vi "HFRR ADV v026 new software.vi"() -> ()   [LabVIEW 2025] (continued)
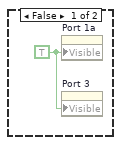
[diagram p3: hidden frame]
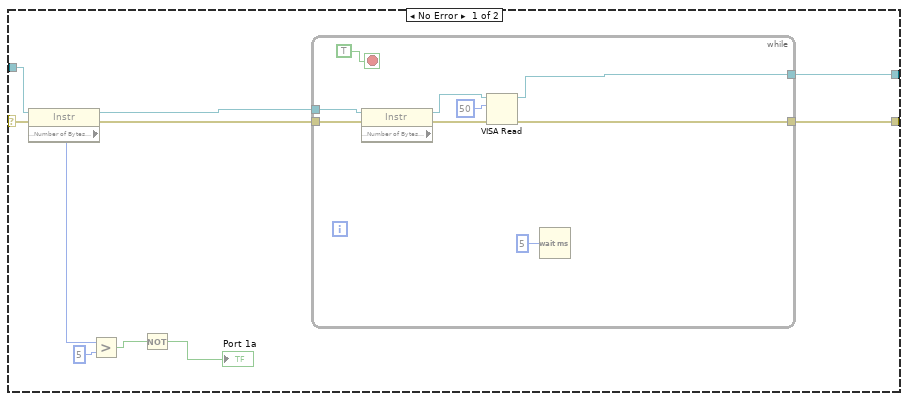
[diagram p4: hidden frame]
            n2893 = call-poly <vilib>:"Append Report Text.vi"("report in"=w3834, "error in (no error)"=w3833) -> ("report out"=w3855:refnum<class "NI_report.lvclass">, "error out"=w3853:errorcluster)  [unwired: 10 in, 2 out]
            n2894 = Concatenate Strings(w3809, w3808, w3807) -> (→"output":string)
            n2895 = call-poly <vilib>:"Append Report Text.vi"("report in"=w3855, "text"=w3808, "error in (no error)"=w3853) -> ("report out"=w3854:refnum<class "NI_report.lvclass">, "error out"=w3852:errorcluster)  [unwired: 9 in, 2 out]
            n2896 = call-dynamic "Print Report.vi"("report in"=w3854, "printer name (default)"=w3862, "error in (no error)"=w3852) -> ("report out"=w3864:refnum<class "NI_report.lvclass">, "error out"=w3865:errorcluster)  [unwired: 11 in]
            n2897 = call-dynamic "Dispose Report.vi"("report in"=w3864, "error in (no error)"=w3865) -> ()  [unwired: 13 in, 1 out]
          }
        }
        n2898 = case shown="True" "Print 2" {
          frame False {
          }
          frame True {
            n2899 = flat-sequence {
              frame #0 {
                n2900 = local read "s.NO"() -> (→"s.NO 2":string)
                n2901 = Wait (ms)(milliseconds to wait=u32 20) -> ()  [unwired: 1 out]
                n2902 = local read "Sample ID  3"() -> (→"Sample ID  6":string)
                n2903 = local read "Sample ID  4"() -> (→"Sample ID  7":string)
                n2904 = local read "Sample ID"() -> (→"Sample ID  2":string)
                n2905 = local read "Tested by"() -> (→"Tested by 2":string)
                n2906 = local read "Test Date"() -> (→"Test Date 2":string)
                n2907 = local read "Humidity after test 3"() -> (→"Humidity after test 4":dbl)
                n2908 = local read "Ref A Test Date :"() -> (→"TITTLE 4":string)
                n2909 = local read "Temperature before test 3"() -> (w3687:dbl)
                n2910 = local read "Temperature before test 3"() -> (→"Temperature after test 5":dbl)
                n2911 = local read "Temperature after test 3"() -> (→"Temperature after test 4":dbl)
                n2912 = local read "Humidity before test 3"() -> (→"Humidity before test 4":dbl)
                n2913 = local write "Temperature before test 3"(w3687) -> ()
                n2914 = local read "image data"() -> (w3678:T15)
                n2915 = String To Path(string="C:\\LAB-IQ\\im\\Temp_resized.jpg") -> (path=w3679:path)
                "path 2" <- w3679
                n2916 = call <vilib>:"Write JPEG File.vi"("image data"=w3678, "path to JPEG file"=w3679) -> ()  [unwired: 8 in, 2 out]
                "Ref A Test Date :" <- "Ref A Test Date :"
                "Ref B Test Date :" <- "Ref B Test Date :"
                "Ref B Scar Value :" <- "Ref B Scar Value :"
                "Ref A Scar Value :" <- "Ref A Scar Value :"
              }
              frame #1 {
                (unwired) HTML_Report_Image_Alignment."MIDDLE" ("alignment (default)")
                w3715 = u16 0 items=["portrait", "landscape"] ("orientation (portrait)")
                (unwired) HTML_Report_Image_Alignment."ABSMIDDLE" ("alignment (default)")
                (unwired) "TESTED BY : "
                (unwired) "TESTED DATE :"
                (unwired) "SAMPLE ID : "
                (unwired) "SAMPLE DESIGN : "
                w3748 = "\r"
                # "add image"
                n2917 = Wait (ms)(milliseconds to wait=u32 20) -> ()  [unwired: 1 out]
                n2918 = local read "Sample ID  2"() -> (w3741:string)
                n2919 = local read "Wear Scar X"() -> (w3713:dbl)
                "Length ( microns ) 2" <- w3713
                n2920 = local read "Wear Scar Y"() -> (w3712:dbl)
                "Wear Scar Y ( microns ) :" <- w3712
                n2921 = local read "Test Date 2"() -> (w3742:string)
                n2922 = local read "Tested by 2"() -> (w3743:string)
                n2923 = local read "String 46"() -> (w3739:string)
                n2924 = local read "String 48"() -> (w3745:string)
                n2925 = local read "String 47"() -> (w3744:string)
                n2926 = local read "String 49"() -> (w3746:string)
                n2927 = local read "String 10"() -> (w3699:string)
                n2928 = local read "s.NO 2"() -> (w3740:string)
                n2929 = Add(x=w3713, y=w3712) -> (x+y=w3711:dbl)
                n2930 = call <vilib>:"New Report.vi"("report type"=enum16{"Standard Report", "HTML"}."HTML") -> ("report out"=w3719:refnum<class "NI_report.lvclass">, "error out"=w3717:errorcluster)  [unwired: 13 in]
                n2931 = Concatenate Strings(w3748, w3739, w3740, w3748, w3745, w3741, w3748, w3744, w3742, w3748, w3746, w3743, w3748) -> (→"test by 2":string)
                n2932 = Concatenate Strings("C:\\LAB-IQ\\Data\\" ("string"), w3699, ".jpg" ("string")) -> ()  [unwired: 1 out]
                n2933 = Divide(x=w3711, y=2.0) -> (x/y=→"Mean Wear ( microns) :":dbl)
                n2934 = call-dynamic "Set Report Orientation.vi"("report in"=w3719, "orientation (portrait)"=w3715, "error in (no error)"=w3717) -> ("report out"=w3718:refnum<class "NI_report.lvclass">, "error out"=w3716:errorcluster)  [unwired: 11 in]
                n2935 = for {
                  N: 5 -> [_]
                  tunnel: w3718 -> [w3769]
                  tunnel: [w3768] -> w3697
                  tunnel: w3716 -> [w3767]
                  tunnel: [w3766] -> w3696
                  n2936 = call-dynamic "Set Report Tab Width.vi"("report in"=w3769, "error in (no error)"=w3767) -> ("report out"=w3768:refnum<class "NI_report.lvclass">, "error out"=w3766:errorcluster)  [unwired: 12 in]
                }
                n2937 = local read "TITTLE"() -> (w3714:string)
                n2938 = call-dynamic "Set Report Header Text.vi"("report in"=w3697, "center header text"=w3714, "error in (no error)"=w3696) -> ("report out"=w3735:refnum<class "NI_report.lvclass">, "error out"=w3734:errorcluster)  [unwired: 11 in]
                n2939 = for {
                  N: 1 -> [_]
                  tunnel: [w3773] -> w3721
                  tunnel: [w3772] -> w3720
                  tunnel: w3735 -> [w3771]
                  tunnel: w3734 -> [w3770]
                  n2940 = call-dynamic "New Report Line.vi"("report in"=w3771, "error in (no error)"=w3770) -> ("report out"=w3773:refnum<class "NI_report.lvclass">, "error out"=w3772:errorcluster)  [unwired: 12 in]
                }
                n2941 = for {
                  N: 2 -> [_]
                  tunnel: [w3765] -> w3727
                  tunnel: [w3764] -> w3726
                  tunnel: w3721 -> [w3763]
                  tunnel: w3720 -> [w3762]
                  n2942 = call-dynamic "New Report Line.vi"("report in"=w3763, "error in (no error)"=w3762) -> ("report out"=w3765:refnum<class "NI_report.lvclass">, "error out"=w3764:errorcluster)  [unwired: 12 in]
                }
                n2943 = for {
                  N: 25 -> [_]
                  tunnel: w3727 -> [w3761]
                  tunnel: w3726 -> [w3759]
                  tunnel: [w3760] -> w3730
                  tunnel: [w3758] -> w3729
                  n2944 = call-dynamic "Set Report Tab Width.vi"("report in"=w3761, "error in (no error)"=w3759) -> ("report out"=w3760:refnum<class "NI_report.lvclass">, "error out"=w3758:errorcluster)  [unwired: 12 in]
                }
                n2945 = control-ref of="Tab Control 9"() -> (w3725:refnum<vi>)
                n2946 = call-dynamic "Append Control Image to Report.vi"("report in"=w3730, "alignment (default)"=HTML_Report_Image_Alignment."ABSMIDDLE", "ctrl reference"=w3725, "error in (no error)"=w3729) -> ("report out"=w3724:refnum<class "NI_report.lvclass">, "error out"=w3723:errorcluster)  [unwired: 8 in, 2 out]
                n2947 = for {
                  N: 3 -> [_]
                  tunnel: [w3757] -> w3708
                  tunnel: [w3756] -> w3707
                  tunnel: w3724 -> [w3755]
                  tunnel: w3723 -> [w3754]
                  n2948 = call-dynamic "New Report Line.vi"("report in"=w3755, "error in (no error)"=w3754) -> ("report out"=w3757:refnum<class "NI_report.lvclass">, "error out"=w3756:errorcluster)  [unwired: 12 in]
                }
                n2949 = for {
                  N: 100 -> [_]
                  tunnel: w3708 -> [w3753]
                  tunnel: w3707 -> [w3751]
                  tunnel: [w3752] -> w3704
                  tunnel: [w3750] -> w3702
                  n2950 = call-dynamic "Set Report Tab Width.vi"("report in"=w3753, "error in (no error)"=w3751) -> ("report out"=w3752:refnum<class "NI_report.lvclass">, "error out"=w3750:errorcluster)  [unwired: 12 in]
                }
                n2951 = String To Path(string="C:\\LAB-IQ\\im\\Temp_resized.jpg") -> (path=w3694:path)
                n2952 = call-poly <vilib>:"Append Image to Report.vi"("report in"=w3704, "path or URL of image"=w3694, "error in (no error)"=w3702) -> ("report out"=w3703:refnum<class "NI_report.lvclass">, "error out"=w3701:errorcluster)  [unwired: 9 in, 2 out]
                n2953 = call-poly <vilib>:"Open HTML Report in Browser.vi"("report in"=w3703, "error in (no error)"=w3701) -> ("report out"=w3738:refnum<class "NI_report.lvclass">, "error out"=w3737:errorcluster)  [unwired: 11 in, 1 out]
                n2954 = call-dynamic "Dispose Report.vi"("report in"=w3738, "error in (no error)"=w3737) -> ()  [unwired: 13 in, 1 out]
              }
              frame #2 {
              }
              frame #3 {
                n2955 = disable-structure shown="Disabled" {
                  frame Disabled {
                    n2956 = local read "String 10"() -> (w3778:string)
                    n2957 = Concatenate Strings("C:\\LAB-IQ-NXT\\Data\\" ("string"), w3778, ".jpg" ("string")) -> (w3776:string)
                    n2958 = String To Path(string=w3776) -> (path=w3775:path)
                    n2959 = Delete(path (use dialog)=w3775) -> ()  [unwired: 4 in, 3 out]
                  }
                  frame Enabled {
                  }
                }
                n2960 = local write "Print 2"(FALSE ("Print")) -> ()
              }
            }
          }
        }
      }
    }
    n2961 = Wait (ms)(milliseconds to wait=u32 50) -> ()  [unwired: 1 out]
    n2962 = Wait (ms)(milliseconds to wait=u32 50) -> ()  [unwired: 1 out]
    n2963 = local read "Quit"() -> (w2123:bool)
  }
  n2964 = VISA Close(VISA resource name=w41, error in (no error)=w40) -> ()  [unwired: 1 out]
  n2965 = while {
    tunnel: [w3938] -> w49
    shift-right: [w3931] -> _
    shift-left: 0.0 -> [w3934]
    shift-right: [w3930] -> _
    shift-left: 0.0 -> [w3933]
    shift-right: [w3929] -> _
    shift-left: 100.0 ("vc_cmd") -> [w3932]
    stop <- w3938 stop-if-true
    # "PID LOGIC"
    n2966 = local read "RUN"() -> (w3936:bool)
    n2967 = local read "Auto Start Temp"() -> (w3925:bool)
    n2968 = local read "Auto Start Test"() -> (w3935:bool)
    n2969 = local read "START TEMP"() -> (w3927:bool)
    n2970 = And(x=w3925, y=w3935) -> (x .and. y?=w3926:bool)
    n2971 = Or(x=w3936, y=w3926) -> (x .or. y?=w3937:bool)
    n2972 = And(x=w3937, y=w3927) -> (x .and. y?=w3928:bool)
    n2973 = Wait (ms)(milliseconds to wait="milliseconds to wait") -> ()  [unwired: 1 out]
    n2974 = case shown="True" w3928 {
      tunnel: [400.0 ("out_vc_cmd") w3958] -> w3929
      tunnel: [w3941 w3960] -> w3930
      tunnel: [w3941 w3959] -> w3931
      tunnel: w3934 -> [_ w3949]
      tunnel: w3933 -> [_ w3948]
      tunnel: w3932 -> [_ w3947]
      frame False {
        w3941 = 0.0 ("error_out")
      }
      frame True {
        n2975 = local read "Set Strk"() -> (w3944:dbl)
        n2976 = local read "LVDT STROKE"() -> (w3942:dbl)
        n2977 = Add(x=w3944, y="Add up Stroke") -> (x+y=w3945:dbl)
        n2978 = formula code="// Zero-Hardcode Explicit Positional-Form PID Engine\n// Inputs: target_stroke, measured_stroke, dt, prev_error, integral_accumulator_in, prev_vc_cmd\n//         kp, ki, kd, max_step_change, max_amplitude, min_amplitude, startup_cmd\n// Outputs: vc_cmd, error_out, out_error, integral_accumulator_out, out_vc_cmd\n\n// 1. Calculate Tracking Error\nfloat current_error = target_stroke - measured_stroke;\nerror_out = current_error;\n\n// 2. Compute Proportional Term\nfloat p_term = kp * current_error;\n\n// 3. Compute Derivative Term\nfloat d_term = 0.0;\nif (dt > 0.0) {\n    d_term = kd * ((current_error - prev_error) / dt);\n}\n\n// 4. Update and Accumulate Integral Term\nfloat current_integral = integral_accumulator_in + (current_error * dt);\nfloat i_term = ki * current_integral;\n\n// 5. Calculate Ideal Target Command\nfloat ideal_command = startup_cmd + p_term + i_term + d_term;\n\n// 6. Anti-Windup Protection (Back-calculation method)\nif (ideal_command > max_amplitude) {\n    float excess = ideal_command - max_amplitude;\n    if (ki > 0.0) {\n        current_integral -= excess / ki;\n    }\n    ideal_command = max_amplitude;\n} else if (ideal_command < min_amplitude) {\n    float excess = ideal_command - min_amplitude;\n    if (ki > 0.0) {\n        current_integral -= excess / ki;\n    }\n    ideal_command = min_amplitude;\n}\n\n// 7. Apply Loop Rate Limiting (Protects voice coil from large voltage steps)\nfloat raw_adjustment = ideal_command - prev_vc_cmd;\n\nif (raw_adjustment > max_step_change) {\n    raw_adjustment = max_step_change;\n} else if (raw_adjustment < -max_step_change) {\n    raw_adjustment = -max_step_change;\n}\n\nfloat next_vc_cmd = prev_vc_cmd + raw_adjustment;\n\n// Final Output Safety Safeguard Clamping\nif (next_vc_cmd > max_amplitude) {\n    next_vc_cmd = max_amplitude;\n} else if (next_vc_cmd < min_amplitude) {\n    next_vc_cmd = min_amplitude;\n}\n\n// 8. Map to Shift Registers for memory persistence\nvc_cmd = next_vc_cmd;\nout_error = current_error;                     \nintegral_accumulator_out = current_integral;  \nout_vc_cmd = next_vc_cmd;"("target_stroke"=w3945, "measured_stroke"=w3942, "dt"="dt", "integral_accumulator_in"=w3948, "prev_error"=w3949, "prev_vc_cmd"=w3947, "kp"="kp", "ki"="ki", "kd"="kd", "max_step_change"="max_step_change", "max_amplitude"="max_amplitude", "min_amplitude"="min_amplitude", "startup_cmd"="startup_cmd") -> ("vc_cmd"=w3964:dbl, "out_error"=w3959:dbl, "integral_accumulator_out"=w3960:dbl, "out_vc_cmd"=w3958:dbl)  [unwired: 1 out]
        "output Vpp" <- w3964
        n2979 = Number To Fractional String(number=w3964, precision (6)=i16 1) -> (F-format string=w3962:string)  [unwired: 2 in]
        n2980 = Concatenate Strings("DAC;" ("string"), w3962) -> (w3946:string)
        n2981 = local write "Due Write"(w3946) -> ()
        "prev_error" <- w3949
        "integral_accumulator_in" <- w3948
        "prev_vc_cmd" <- w3947
      }
    }
    n2982 = local read "Quit"() -> (w3938:bool)
  }
  n2983 = Or(x=w45, y=w44) -> (x .or. y?=w46:bool)
  n2984 = Or(x=w42, y=w46) -> (x .or. y?=w51:bool)
  n2985 = control-ref of="new picture"() -> ()  [unwired: 1 out]
  n2986 = Or(x=w54, y=w51) -> (x .or. y?=w48:bool)
  n2987 = Or(x=w48, y=w49) -> (x .or. y?=w43:bool)
  n2988 = while {
    tunnel: [w3965] -> w53
    i -> [w3972]
    stop <- w3965 stop-if-true
    n2989 = local read "Quit"() -> (w3965:bool)
    n2990 = Equal To 0?(x=w3972) -> (x = 0?=w3970:bool)
    n2991 = call "Elapsed Time3"("Time Target (s)"=45.0, "Auto Reset"=TRUE) -> ("Time has Elapsed"=w3969:bool)  [unwired: 10 in, 7 out]
    n2992 = Wait (ms)(milliseconds to wait=u32 50) -> ()  [unwired: 1 out]
    n2993 = Or(x=w3969, y=w3970) -> (x .or. y?=w3971:bool)
    n2994 = case shown="True" w3971 {
      frame False {
      }
      frame True {
        n2995 = call <vilib>:"System Exec.vi"("run minimized? (F)"=TRUE, "error in (no error)"="error in (no error)", "command line"="powercfg.exe -change -monitor-timeout-ac 0") -> ("error out"=w3983:errorcluster)  [unwired: 5 in, 3 out]
        n2996 = call <vilib>:"System Exec.vi"("run minimized? (F)"=TRUE, "error in (no error)"=w3983, "command line"="powercfg.exe -change -disk-timeout-ac 0") -> ("error out"=w3982:errorcluster)  [unwired: 5 in, 3 out]
        n2997 = call <vilib>:"System Exec.vi"("run minimized? (F)"=TRUE, "error in (no error)"=w3982, "command line"="powercfg.exe -change -standby-timeout-ac 0") -> ("error out"=w3981:errorcluster)  [unwired: 5 in, 3 out]
        n2998 = call <vilib>:"System Exec.vi"("run minimized? (F)"=TRUE, "error in (no error)"=w3981, "command line"="powercfg.exe -change -hibernate-timeout-ac 0") -> ("error out"=w3980:errorcluster)  [unwired: 5 in, 3 out]
        n2999 = call <vilib>:"Simple Error Handler.vi"("error in (no error)"=w3980) -> ("error out"=w3986:errorcluster)  [unwired: 4 in, 4 out]
        n3000 = call <vilib>:"Clear Errors.vi"("error in (no error)"=w3986) -> ("error out"=→"error out":errorcluster)  [unwired: 5 in, 1 out]
      }
    }
  }
  n3001 = Compound Arithmetic op=OR(w56, w43, w53) -> (w55:bool)
  n3002 = flat-sequence {
    tunnel: w55 -> [_]
    tunnel: [w3988] -> w25
    tunnel: w25 -> [_]
    frame #0 {
      n3003 = call "CLOSE CONNECTION.vi"() -> ("error out"=w3988:errorcluster)  [unwired: 11 in]
    }
    frame #1 {
      n3004 = Quit LabVIEW(quit? (T)=TRUE) -> ()
      n3005 = local write "Quit"(FALSE ("EXIT")) -> ()
    }
  }
  n3006 = property on="Heater Button" class="Bool (strict)"("Visible"=TRUE) -> ()  [unwired: 2 in, 2 out]
  n3007 = while {
    tunnel: [w3995] -> _
    i -> [w3995]
    stop <- w3991 stop-if-true
    # "Langauage selection"
    n3008 = Equal?(x="Lan flag", y=22.0) -> ()  [unwired: 1 out]
    n3009 = disable-structure shown="Disabled" {
      frame Disabled {
        n3010 = stacked-sequence {
          frame #0 {
            n3011 = case shown="\"Russian\"" "Language Selection" {
              tunnel: [0 1] -> w3997
              frame "English", Default {
              }
              frame "Russian" {
              }
            }
            n3012 = for {
              N: 130 -> [_]
              tunnel: "Table" -> [w4006]
              tunnel: w3997 -> [w4005]
              i -> [w4004]
              n3013 = Index Array(array=w4006, index (row)=w4004, index (col)=w4005) -> (element=w4003:string)
              n3014 = case shown="1" w4004 {
                tunnel: w4003 -> [w4007 w4008 _ w4009 w4010 w4011 w4012 w4013 w4014 w4015 w4016 w4017 w4018 w4019 w4020 w4021 w4022 w4023 w4024 w4025 w4026 w4027 w4028 w4029 w4030 w4031 w4032 w4033 w4034 _ _ w4035 w4036 w4037 w4038 w4039 w4040 w4049 w4056 w4063 w4070 w4074 w4077 w4080 w4082 w4084 w4085 w4086 w4087 w4088 w4089 w4090 w4091 w4092 w4093 w4094 w4095 w4096 w4097 w4098 w4099 w4100 w4101 w4102 w4103 w4104 w4105 w4106 w4107 w4108 w4109 w4110 w4111 w4112 w4113 w4114 w4115 w4116 w4117 w4118 w4119 w4120 w4121 w4122 w4123 w4124 w4125 w4126 w4127 w4128 w4129 w4130 w4131 w4132 w4133 w4134 w4135 w4136 w4137 w4138 w4139 w4140 w4141 w4142 w4143 _ w4144 w4145 w4146 w4147 w4148 w4149 w4150 w4151 w4152 w4153 w4154 w4155 w4156 _ w4157 w4158 w4159 w4160 w4161 w4162 _]
                frame 0 {
                  n3015 = local write "S"(w4007) -> ()
                }
                frame 1 {
                  n3016 = local write "S 2"(w4008) -> ()
                }
                frame 2 {
                }
                frame 3 {
                  n3017 = local write "S 4"(w4009) -> ()
                }
                frame 4 {
                  n3018 = property on="FILE" class="Str"("Caption.Text"=w4010) -> ()  [unwired: 2 in, 2 out]
                }
                frame 5 {
                  n3019 = property on="Fuel Discription :" class="Str"("Caption.Text"=w4011) -> ()  [unwired: 2 in, 2 out]
                }
                frame 6 {
                  n3020 = property on="Remarks :" class="Str"("Caption.Text"=w4012) -> ()  [unwired: 2 in, 2 out]
                }
                frame 7 {
                  n3021 = property on="Save & Continue" class="Bool (strict)"("Boolean Text.Text"=w4013) -> ()  [unwired: 2 in, 2 out]
                }
                frame 8 {
                }
                frame 9 {
                  n3022 = property on="Set Hz" class="DigNum (strict)"("Caption.Text"=w4015) -> ()  [unwired: 2 in, 2 out]
                }
                frame 10 {
                }
                frame 11 {
                  n3023 = property on="NORMAL LOAD" class="DigNum (strict)"("Caption.Text"=w4017) -> ()  [unwired: 2 in, 2 out]
                }
                frame 12 {
                }
                frame 13 {
                  n3024 = property on="Set Temp" class="DigNum (strict)"("Caption.Text"=w4019) -> ()  [unwired: 2 in, 2 out]
                }
                frame 14 {
                  n3025 = local write "S 15"(w4020) -> ()
                }
                frame 15 {
                  n3026 = property on="Set Rh" class="DigNum (strict)"("Caption.Text"=w4021) -> ()  [unwired: 2 in, 2 out]
                }
                frame 16 {
                }
                frame 17 {
                  n3027 = local write "S 18"(w4023) -> ()
                }
                frame 18 {
                  "String 17" <- w4024
                }
                frame 19 {
                  n3028 = property on="test time" class="DigNum (strict)"("Caption.Text"=w4025) -> ()  [unwired: 2 in, 2 out]
                }
                frame 20 {
                  "String 18" <- w4026
                  "String 22" <- w4026
                }
                frame 21 {
                  n3029 = property on="Elapsed time" class="DigNum (strict)"("Caption.Text"=w4027) -> ()  [unwired: 2 in, 2 out]
                }
                frame 22 {
                  n3030 = property on="Samplingtime 2" class="DigNum (strict)"("Caption.Text"=w4028) -> ()  [unwired: 2 in, 2 out]
                }
                frame 23 {
                  "String 21" <- w4029
                }
                frame 24 {
                  n3031 = property on="Countdown" class="DigNum (strict)"("Caption.Text"=w4030) -> ()  [unwired: 2 in, 2 out]
                }
                frame 25 {
                  n3032 = property on="Countdown 2" class="DigNum (strict)"("Caption.Text"=w4031) -> ()  [unwired: 2 in, 2 out]
                }
                frame 26 {
                  n3033 = property on="Engage" class="Bool (strict)"("Boolean Text.Text"=w4032) -> ()  [unwired: 2 in, 2 out]
                }
                frame 27 {
                  n3034 = property on="Boolean  4" class="Bool (strict)"("Boolean Text.Text"=w4033) -> ()  [unwired: 2 in, 2 out]
                }
                frame 28 {
                  n3035 = property on="Test \nStatus" class="Bool (strict)"("Boolean Text.Text"=w4034) -> ()  [unwired: 2 in, 2 out]
                }
                frame 29 {
                }
                frame 30 {
                }
                frame 31 {
                }
                frame 32 {
                  n3036 = property on="RSTCOF" class="Bool"("Boolean Text.Text"=w4036) -> ()  [unwired: 2 in, 2 out]
                  n3037 = property on="RST FF" class="Bool"("Boolean Text.Text"=w4036) -> ()  [unwired: 2 in, 2 out]
                  n3038 = property on="RST TEMP" class="Bool"("Boolean Text.Text"=w4036) -> ()  [unwired: 2 in, 2 out]
                  n3039 = property on="RSTV1 3" class="Bool"("Boolean Text.Text"=w4036) -> ()  [unwired: 2 in, 2 out]
                  n3040 = property on="rstv2" class="Bool"("Boolean Text.Text"=w4036) -> ()  [unwired: 2 in, 2 out]
                  n3041 = property on="RSTV1 2" class="Bool"("Boolean Text.Text"=w4036) -> ()  [unwired: 2 in, 2 out]
                  n3042 = property on="RST CP" class="Bool"("Boolean Text.Text"=w4036) -> ()  [unwired: 2 in, 2 out]
                }
                frame 33 {
                  "S 61" <- w4037
                }
                frame 34 {
                  "String 23" <- w4038
                }
                frame 35 {
                  n3043 = property on="Rh Before" class="DigNum (strict)"("Caption.Text"=w4039) -> ()  [unwired: 2 in, 2 out]
                }
                frame 36 {
                  n3044 = Match Pattern(string=w4040, regular expression=",") -> (before substring=→"bs":string, after substring=→"as":string)  [unwired: 1 in, 2 out]
                  n3045 = property on="Rh After" class="DigNum (strict)"("Caption.Text"=w4040) -> ()  [unwired: 2 in, 2 out]
                }
                frame 37 {
                  n3046 = Match Pattern(string=w4049, regular expression=",") -> (before substring=w4048:string, after substring=w4047:string)  [unwired: 1 in, 2 out]
                  "bs" <- w4048
                  "as" <- w4047
                  n3047 = Concatenate Strings(w4048, w4047) -> (w4044:string)
                  n3048 = property on="Humidity before test 2" class="DigNum (strict)"("Caption.Text"=w4044) -> ()  [unwired: 2 in, 2 out]
                  n3049 = Concatenate Strings(w4044, "=" ("string")) -> (w4045:string)
                  n3050 = local write "S 38"(w4045) -> ()
                }
                frame 38 {
                  n3051 = Match Pattern(string=w4056, regular expression=",") -> (before substring=w4055:string, after substring=w4054:string)  [unwired: 1 in, 2 out]
                  "bs" <- w4055
                  "as" <- w4054
                  n3052 = Concatenate Strings(w4055, w4054) -> (w4051:string)
                  n3053 = property on="Humidity after test 2" class="DigNum (strict)"("Caption.Text"=w4051) -> ()  [unwired: 2 in, 2 out]
                  n3054 = Concatenate Strings(w4051, "=" ("string")) -> (w4053:string)
                  n3055 = local write "S 39"(w4053) -> ()
                }
                frame 39 {
                  n3056 = Match Pattern(string=w4063, regular expression=",") -> (before substring=w4062:string, after substring=w4061:string)  [unwired: 1 in, 2 out]
                  "bs" <- w4062
                  "as" <- w4061
                  n3057 = Concatenate Strings(w4062, w4061) -> (w4058:string)
                  n3058 = property on="Temperature before test 2" class="DigNum (strict)"("Caption.Text"=w4058) -> ()  [unwired: 2 in, 2 out]
                  n3059 = Concatenate Strings(w4058, "=" ("string")) -> (→"String 34":string)
                }
                frame 40 {
                  n3060 = Match Pattern(string=w4070, regular expression=",") -> (before substring=w4069:string, after substring=w4068:string)  [unwired: 1 in, 2 out]
                  "bs" <- w4069
                  "as" <- w4068
                  n3061 = Concatenate Strings(w4069, w4068) -> (w4065:string)
                  n3062 = property on="Temperature after test 2" class="DigNum (strict)"("Caption.Text"=w4065) -> ()  [unwired: 2 in, 2 out]
                  n3063 = Concatenate Strings(w4065, "=" ("string")) -> (→"String 35":string)
                  n3064 = property on="Temperature after test" class="DigNum (strict)"("Caption.Text"=w4065) -> ()  [unwired: 2 in, 2 out]
                }
                frame 41 {
                  n3065 = property on="AVP 2" class="DigNum (strict)"("Caption.Text"=w4074) -> ()  [unwired: 2 in, 2 out]
                  n3066 = Concatenate Strings(w4074, "=" ("string")) -> (→"String 36":string)
                }
                frame 42 {
                  n3067 = property on="MWSD 2" class="DigNum (strict)"("Caption.Text"=w4077) -> ()  [unwired: 2 in, 2 out]
                  n3068 = Concatenate Strings(w4077, "=" ("string")) -> (→"String 37":string)
                }
                frame 43 {
                  n3069 = property on="HCF 2" class="DigNum (strict)"("Caption.Text"=w4080) -> ()  [unwired: 2 in, 2 out]
                  n3070 = Concatenate Strings(w4080, "=" ("string")) -> (→"String 38":string)
                }
                frame 44 {
                  n3071 = Concatenate Strings(w4082, "=" ("string")) -> (→"String 39":string)
                  n3072 = property on="WS1.4 2" class="DigNum (strict)"("Caption.Text"=w4082) -> ()  [unwired: 2 in, 2 out]
                }
                frame 45 {
                }
                frame 46 {
                  n3073 = local write "S 47"(w4085) -> ()
                }
                frame 47 {
                  n3074 = local write "S 48"(w4086) -> ()
                }
                frame 48 {
                  n3075 = local write "S 49"(w4087) -> ()
                }
                frame 49 {
                  n3076 = local write "S 50"(w4088) -> ()
                }
                frame 50 {
                  n3077 = local write "S 51"(w4089) -> ()
                }
                frame 51 {
                  n3078 = local write "S 52"(w4090) -> ()
                }
                frame 52 {
                  n3079 = local write "S 53"(w4091) -> ()
                }
                frame 53 {
                  n3080 = local write "S 54"(w4092) -> ()
                }
                frame 54 {
                  n3081 = local write "S 55"(w4093) -> ()
                }
                frame 55 {
                  n3082 = local write "S 56"(w4094) -> ()
                }
                frame 56 {
                  n3083 = local write "S 57"(w4095) -> ()
                }
                frame 57 {
                  n3084 = local write "S 58"(w4096) -> ()
                }
                frame 58 {
                  n3085 = local write "S 59"(w4097) -> ()
                }
                frame 59 {
                  n3086 = local write "S 60"(w4098) -> ()
                }
                frame 60 {
                  n3087 = local write "S 62"(w4099) -> ()
                }
                frame 61 {
                  n3088 = local write "S 63"(w4100) -> ()
                }
                frame 62 {
                  n3089 = local write "S 64"(w4101) -> ()
                }
                frame 63 {
                  n3090 = local write "S 65"(w4102) -> ()
                }
                frame 64 {
                  n3091 = local write "S 66"(w4103) -> ()
                }
                frame 65 {
                  n3092 = local write "S 67"(w4104) -> ()
                }
                frame 66 {
                  n3093 = local write "S 68"(w4105) -> ()
                }
                frame 67 {
                  n3094 = local write "S 69"(w4106) -> ()
                }
                frame 68 {
                  n3095 = local write "S 70"(w4107) -> ()
                }
                frame 69 {
                  n3096 = local write "S 71"(w4108) -> ()
                }
                frame 70 {
                  n3097 = local write "S 72"(w4109) -> ()
                }
                frame 71 {
                  n3098 = local write "S 73"(w4110) -> ()
                }
                frame 72 {
                  n3099 = local write "S 74"(w4111) -> ()
                }
                frame 73 {
                  n3100 = local write "S 75"(w4112) -> ()
                }
                frame 74 {
                  n3101 = local write "S 76"(w4113) -> ()
                }
                frame 75 {
                  n3102 = local write "S 77"(w4114) -> ()
                }
                frame 76 {
                  n3103 = local write "S 78"(w4115) -> ()
                }
                frame 77 {
                  n3104 = local write "S 79"(w4116) -> ()
                }
                frame 79 {
                  n3105 = property on="Sample Temperature ( °C )" class="XYGraph (strict)"("Y Scale.Name Label.Text"=w4117) -> ()  [unwired: 2 in, 2 out]
                }
                frame 80 {
                  n3106 = local write "S 81"(w4118) -> ()
                  n3107 = property on="Humidity ( %RH )" class="XYGraph (strict)"("Y Scale.Name Label.Text"=w4118) -> ()  [unwired: 2 in, 2 out]
                }
                frame 78 {
                  n3108 = property on="Air Temperature  ( °C )" class="XYGraph (strict)"("X Scale.Name Label.Text"=w4119) -> ()  [unwired: 2 in, 2 out]
                  n3109 = property on="Humidity ( %RH )" class="XYGraph (strict)"("X Scale.Name Label.Text"=w4119) -> ()  [unwired: 2 in, 2 out]
                  n3110 = property on="Sample Temperature ( °C )" class="XYGraph (strict)"("X Scale.Name Label.Text"=w4119) -> ()  [unwired: 2 in, 2 out]
                  n3111 = property on="Coefficient Of Friction" class="XYGraph (strict)"("X Scale.Name Label.Text"=w4119) -> ()  [unwired: 2 in, 2 out]
                }
                frame 81 {
                  n3112 = property on="Air Temperature  ( °C )" class="XYGraph (strict)"("Y Scale.Name Label.Text"=w4120) -> ()  [unwired: 2 in, 2 out]
                }
                frame 82 {
                  n3113 = local write "S 84"(w4121) -> ()
                }
                frame 83 {
                  n3114 = local write "S 85"(w4122) -> ()
                }
                frame 84 {
                  n3115 = local write "S 86"(w4123) -> ()
                }
                frame 85 {
                  n3116 = local write "S 87"(w4124) -> ()
                }
                frame 86 {
                  n3117 = local write "S 88"(w4125) -> ()
                }
                frame 87 {
                }
                frame 88 {
                  n3118 = local write "S 90"(w4127) -> ()
                }
                frame 89 {
                  n3119 = local write "S 91"(w4128) -> ()
                }
                frame 90 {
                  n3120 = local write "S 92"(w4129) -> ()
                }
                frame 91 {
                  n3121 = local write "S 93"(w4130) -> ()
                }
                frame 92 {
                  n3122 = local write "S 94"(w4131) -> ()
                }
                frame 93 {
                  n3123 = local write "S 95"(w4132) -> ()
                }
                frame 94 {
                  n3124 = local write "S 96"(w4133) -> ()
                }
                frame 95 {
                  n3125 = local write "S 97"(w4134) -> ()
                }
                frame 96 {
                  n3126 = local write "S 98"(w4135) -> ()
                }
                frame 97 {
                  n3127 = local write "S 99"(w4136) -> ()
                }
                frame 98 {
                  n3128 = local write "S 100"(w4137) -> ()
                }
                frame 99 {
                  n3129 = local write "S 101"(w4138) -> ()
                }
                frame 100 {
                  n3130 = local write "S 102"(w4139) -> ()
                }
                frame 101 {
                  n3131 = local write "S 103"(w4140) -> ()
                }
                frame 102 {
                  n3132 = local write "S 104"(w4141) -> ()
                }
                frame 103 {
                  n3133 = local write "S 105"(w4142) -> ()
                }
                frame 104 {
                  n3134 = local write "S 106"(w4143) -> ()
                }
                frame 105 {
                }
                frame 106 {
                  n3135 = property on="OK Button 17" class="Bool (strict)"("Boolean Text.Text"=w4144) -> ()  [unwired: 2 in, 2 out]
                }
                frame 107 {
                  n3136 = property on="OK Button 16" class="Bool (strict)"("Boolean Text.Text"=w4145) -> ()  [unwired: 2 in, 2 out]
                }
                frame 108 {
                  n3137 = property on="TITTLE" class="Str"("Caption.Text"=w4146) -> ()  [unwired: 2 in, 2 out]
                }
                frame 109 {
                  "String 30" <- w4147
                }
                frame 110 {
                  n3138 = property on="Test Date" class="Str"("Caption.Text"=w4148) -> ()  [unwired: 2 in, 2 out]
                  "String 31" <- w4148
                }
                frame 111 {
                  n3139 = property on="Sample ID" class="Str"("Caption.Text"=w4149) -> ()  [unwired: 2 in, 2 out]
                  "String 32" <- w4149
                }
                frame 112 {
                  n3140 = property on="Tested by" class="Str"("Caption.Text"=w4150) -> ()  [unwired: 2 in, 2 out]
                  "String 33" <- w4150
                }
                frame 113 {
                  n3141 = property on="System Configured Printers 2" class="Arr (strict)"("Caption.Text"=w4151) -> ()  [unwired: 2 in, 2 out]
                }
                frame 114 {
                  n3142 = property on="Selected Printer" class="Str"("Caption.Text"=w4152) -> ()  [unwired: 2 in, 2 out]
                }
                frame 115 {
                  n3143 = property on="Select Printer 3" class="DigNum (strict)"("Caption.Text"=w4153) -> ()  [unwired: 2 in, 2 out]
                }
                frame 116 {
                  n3144 = property on="Print" class="Bool (strict)"("Boolean Text.Text"=w4154) -> ()  [unwired: 2 in, 2 out]
                }
                frame 117 {
                  "String 41" <- w4155
                }
                frame 118 {
                  n3145 = property on="tested by" class="Str"("Caption.Text"=w4156) -> ()  [unwired: 2 in, 2 out]
                }
                frame 119 {
                }
                frame 120 {
                  n3146 = property on="Export" class="Bool (strict)"("Boolean Text.Text"=w4157) -> ()  [unwired: 2 in, 2 out]
                }
                frame 121 {
                }
                frame 122 {
                }
                frame 123 {
                  n3147 = property on="Select File Type" class="Enum (strict)"("Caption.Text"=w4160) -> ()  [unwired: 2 in, 2 out]
                }
                frame 124 {
                  n3148 = property on="s.NO" class="Str"("Caption.Text"=w4161) -> ()  [unwired: 2 in, 2 out]
                  "String 45" <- w4161
                }
                frame 125 {
                  n3149 = property on="trip1 8" class="Bool (strict)"("Boolean Text.Text"=w4162) -> ()  [unwired: 2 in, 2 out]
                }
                frame 126, Default {
                }
              }
            }
          }
          frame #1 {
            w4170 = TRUE ("Visible")
            n3150 = local read "S 91"() -> (w4187:string)
            n3151 = local read "S 90"() -> (w4186:string)
            n3152 = local read "S 88"() -> (w4185:string)
            n3153 = property on="File Path" class="Path"("Caption.Text"=w4186) -> ()  [unwired: 2 in, 2 out]
            n3154 = local read "S 71"() -> (w4180:string)
            n3155 = local read "S 86"() -> (w4182:string)
            n3156 = local read "S 85"() -> (w4183:string)
            n3157 = local read "S 87"() -> (w4181:string)
            n3158 = local read "S 84"() -> (w4184:string)
            n3159 = local read "S 103"() -> (w4169:string)
            n3160 = local read "S 104"() -> (w4168:string)
            n3161 = property on="Password" class="Str"("Caption.Text"=w4183) -> ()  [unwired: 2 in, 2 out]
            n3162 = property on="EDIT" class="Bool (strict)"("Boolean Text.Text"=w4180) -> ()  [unwired: 2 in, 2 out]
            n3163 = property on="SAVE" class="Bool (strict)"("Boolean Text.Text"=w4184) -> ()  [unwired: 2 in, 2 out]
            n3164 = Build Array(w4169, w4168) -> (w4167:string[])
            n3165 = property on="Heater Button" class="Bool (strict)"("Strings [4]"=w4167) -> ()  [unwired: 2 in, 2 out]
            n3166 = local read "S 92"() -> (w4179:string)
            n3167 = local read "S 93"() -> (w4178:string)
            n3168 = local read "S 105"() -> (w4165:string)
            n3169 = local read "S 106"() -> (w4164:string)
            n3170 = Build Array(w4179, w4178) -> ()  [unwired: 1 out]
            n3171 = Build Array(w4165, w4164) -> (w4166:string[])
            n3172 = local read "S 95"() -> (w4176:string)
            n3173 = local read "S 94"() -> (w4177:string)
            n3174 = local read "bs"() -> (w4192:string)
            n3175 = local read "as"() -> (w4193:string)
            n3176 = property on="Humidity" class="Bool (strict)"("Strings [4]"=w4166) -> ()  [unwired: 2 in, 2 out]
            n3177 = Concatenate Strings(w4192, "\r", w4193) -> ()  [unwired: 1 out]
            n3178 = property on="Rh After" class="DigNum (strict)"("Caption.Size to Text?"=TRUE ("Caption.Size to Text")) -> ()  [unwired: 2 in, 2 out]
            n3179 = local read "S 48"() -> (w4216:string)
            n3180 = local read "S 50"() -> (w4214:string)
            n3181 = local read "S 51"() -> (w4213:string)
            n3182 = local read "S 49"() -> (w4215:string)
            n3183 = local read "S 52"() -> (w4212:string)
            n3184 = local read "as"() -> (w4197:string)
            n3185 = local read "bs"() -> (w4198:string)
            n3186 = local read "S 56"() -> (w4211:string)
            n3187 = local read "S 57"() -> (w4210:string)
            n3188 = local read "S 58"() -> (w4209:string)
            n3189 = local read "S 59"() -> (w4208:string)
            n3190 = property on="OPEN" class="Bool (strict)"("Boolean Text.Text"=w4212) -> ()  [unwired: 2 in, 2 out]
            n3191 = property on="OPEN 1" class="Bool (strict)"("Boolean Text.Text"=w4216) -> ()  [unwired: 2 in, 2 out]
            n3192 = property on="OPEN 2" class="Bool (strict)"("Boolean Text.Text"=w4215) -> ()  [unwired: 2 in, 2 out]
            n3193 = property on="OPEN 3" class="Bool (strict)"("Boolean Text.Text"=w4214) -> ()  [unwired: 2 in, 2 out]
            n3194 = property on="OPEN 4" class="Bool (strict)"("Boolean Text.Text"=w4213) -> ()  [unwired: 2 in, 2 out]
            n3195 = Concatenate Strings(w4198, "\r", w4197) -> ()  [unwired: 1 out]
            n3196 = local read "S 102"() -> (w4171:string)
            n3197 = property on="КОФ1" class="DigNum (strict)"("Caption.Text"=w4211) -> ()  [unwired: 2 in, 2 out]
            n3198 = local read "S 98"() -> (w4175:string)
            n3199 = local read "S 99"() -> (w4174:string)
            n3200 = local read "S 100"() -> (w4173:string)
            n3201 = local read "S 101"() -> (w4172:string)
            n3202 = property on="КОФ2" class="DigNum (strict)"("Caption.Text"=w4210) -> ()  [unwired: 2 in, 2 out]
            n3203 = property on="КОФ3" class="DigNum (strict)"("Caption.Text"=w4209) -> ()  [unwired: 2 in, 2 out]
            n3204 = property on="КОФ4" class="DigNum (strict)"("Caption.Text"=w4208) -> ()  [unwired: 2 in, 2 out]
            n3205 = local read "bs"() -> (w4196:string)
            n3206 = local read "as"() -> (w4195:string)
            n3207 = local read "S 60"() -> (w4207:string)
            n3208 = local read "S 54"() -> (w4217:string)
            n3209 = Concatenate Strings(w4196, "\r", w4195) -> ()  [unwired: 1 out]
            n3210 = Concatenate Strings(w4217, w4207) -> ()  [unwired: 1 out]
            n3211 = local read "S 77"() -> (→"String 43":string)
            n3212 = local read "S 76"() -> (w4190:string)
            n3213 = local read "S 78"() -> (w4189:string)
            n3214 = local read "S 71"() -> (w4201:string)
            n3215 = local read "S 66"() -> (w4206:string)
            n3216 = local read "S 67"() -> (w4205:string)
            n3217 = local read "S 68"() -> (w4204:string)
            n3218 = local read "S 69"() -> (w4203:string)
            n3219 = local read "S 70"() -> (w4202:string)
            n3220 = property on="AIR TEMP" class="DigNum (strict)"("Caption.Text"=w4189) -> ()  [unwired: 2 in, 2 out]
            n3221 = property on="Set Strk" class="DigNum (strict)"("Caption.Text"=w4190) -> ()  [unwired: 2 in, 2 out]
            n3222 = property on="SPEED OUT:" class="DigNum (strict)"("Caption.Text"=w4204) -> ()  [unwired: 2 in, 2 out]
            n3223 = property on="EDIT" class="Bool (strict)"("Boolean Text.Text"=w4201) -> ()  [unwired: 2 in, 2 out]
            n3224 = local read "S 79"() -> (w4188:string)
          }
          frame #2 {
          }
        }
        n3225 = local write "Lan flag"(10.0 ("Lan flag")) -> ()
      }
      frame Enabled {
      }
    }
    n3226 = Wait (ms)(milliseconds to wait=u32 2000) -> ()  [unwired: 1 out]
    n3227 = local read "Quit"() -> (w3991:bool)
  }
  n3228 = while {
    shift-right: [w4223] -> _
    shift-left: _ -> [w4224]
    shift-right: [w4221] -> _
    shift-left: T17 {"Read Heave and Surge"="", "Bytes at Heave Port"=0.0, "Heave and Surge COM Port:"="COM9", "Com Port 2"="COM7", "Residual Due"="", "Heave COM Status 2"=TRUE, "Heave COM Status"=TRUE, "Port 2"=TRUE, "Sway PPR"=6400.0, "Surge PPR"=6400.0, "Heave PPR"=6400.0, "Sway Pitch"=2.0, "Surge Pitch"=3.0, "Heave Pitch"=4.0, "Sway Pulses/mm"=320.0, "Surge Pulses/mm"=1600.0, "Heave Pulses/mm"=1600.0, "inner loop"=0.0, "Read Heave and Surge 2"="", "String 36"="", "Write S"=FALSE, "WriteCC1"=[""], "Heave COM Loop"=0, "LastCom"="", "EXIT"=FALSE, "Error Heave"={"status"=TRUE, "code"=-1073807343, "source"=""}} -> [w4220]
    shift-right: [w4218] -> _
    shift-left: enum16{"init", "MAIN", "Panel Close"}."init" -> [w4219]
    stop <- w4222 stop-if-true
    # "HUMIDITY LOOP LOGIC"
    n3229 = case shown="\"MAIN\"" w4219 {
      tunnel: w4224 -> [w4238 w4255 w4312 w4314]
      tunnel: [w4233 w4260 w4312 w4314] -> w4223
      tunnel: [_ _ TRUE _] -> w4222
      tunnel: [w4230 w4258 w4310 w4313] -> w4221
      tunnel: w4220 -> [w4235 w4254 w4310 w4313]
      tunnel: [enum16{"init", "MAIN", "Panel Close"}."MAIN" w4249 _ _] -> w4218
      frame "init" {
        n3230 = local read "Com Port 1"() -> (w4227:refnum<visa-resource-name>)
        n3231 = Bundle By Name(cluster=w4235, "Heave and Surge COM Port:"=w4227) -> (w4234:T17)
        n3232 = call "Instrument fgv uno.vi"("Enum"=T28."INIT", "error in (no error) 2"=w4238, "INPUT"=w4234) -> ("error"=w4236:errorcluster, "output"=w4232:T17)  [unwired: 6 in, 1 out]
        n3233 = case shown="Error" w4236 {
          selector: w4236 -> [w4240 _]
          tunnel: [w4240 w4244] -> w4233
          tunnel: w4232 -> [w4239 w4242]
          tunnel: [w4239 w4241] -> w4231
          frame No Error {
          }
          frame Error {
            n3234 = call "Instrument fgv uno.vi"("Enum"=T28."ERROR INIT", "INPUT"=w4242) -> ("error"=w4245:errorcluster, "output"=w4241:T17)  [unwired: 7 in, 1 out]
            n3235 = call <vilib>:"Clear Errors.vi"("error in (no error)"=w4245) -> ("error out"=w4244:errorcluster)  [unwired: 5 in, 1 out]
          }
        }
        n3236 = local read "LastCom Humidity"() -> (w4226:string)
        n3237 = Unbundle By Name(w4231) -> ("Heave COM Status 2"=→"COM Status":bool, "Error Heave"=→"Error  2":errorcluster)  [unwired: 1 out]
        n3238 = Bundle By Name(cluster=w4231, "LastCom"=w4226) -> (w4230:T17)
      }
      frame "MAIN" {
        n3239 = Unbundle By Name(w4254) -> ("Com Port 2"=w4262:refnum<visa-resource-name>)
        n3240 = local read "Com Port 1"() -> (w4248:refnum<visa-resource-name>)
        n3241 = local write "Com Port 5"(w4262) -> ()
        n3242 = Bundle By Name(cluster=w4254, "Heave and Surge COM Port:"=w4248) -> (w4253:T17)
        n3243 = Equal?(x=w4262, y=w4248) -> (x = y?=w4261:bool)
        n3244 = case shown="True" w4261 {
          tunnel: [w4266 w4283] -> w4260
          tunnel: w4255 -> [w4267 w4289]
          tunnel: w4253 -> [w4265 w4287]
          tunnel: [w4264 w4282] -> w4258
          frame False {
            n3245 = call <vilib>:"Clear Errors.vi"("error in (no error)"=w4267) -> ("error out"=w4263:errorcluster)  [unwired: 5 in, 1 out]
            n3246 = call "Instrument fgv uno.vi"("Enum"=T28."ERROR INIT", "error in (no error) 2"=w4263, "INPUT"=w4265) -> ("error"=w4269:errorcluster, "output"=w4264:T17)  [unwired: 6 in, 1 out]
            n3247 = call <vilib>:"Clear Errors.vi"("error in (no error)"=w4269) -> ("error out"=w4266:errorcluster)  [unwired: 5 in, 1 out]
          }
          frame True {
            n3248 = call "Instrument fgv uno.vi"("Enum"=T28."READ", "error in (no error) 2"=w4289, "INPUT"=w4287) -> ("error"=w4288:errorcluster, "output"=w4280:T17)  [unwired: 6 in, 1 out]
            n3249 = Bundle By Name(cluster=w4280, "String 36"="WRITE HUMIDITY") -> (w4279:T17)
            n3250 = case shown="True" "Write" {
              selector: "Write" -> [_ w4309]
              tunnel: w4288 -> [w4302 w4308]
              tunnel: [w4302 w4307] -> w4277
              tunnel: w4279 -> [w4301 w4304]
              tunnel: [w4301 w4303] -> w4276
              frame False {
              }
              frame True {
                n3251 = Not(x=w4309) -> (.not. x?=w4305:bool)
                n3252 = local write "Write"(w4305) -> ()
                n3253 = call "Instrument fgv uno.vi"("Enum"=T28."MANUAL WRITE", "error in (no error) 2"=w4308, "INPUT"=w4304) -> ("error"=w4307:errorcluster, "output"=w4303:T17)  [unwired: 6 in, 1 out]
              }
            }
            n3254 = Array Size(array="WriteHumidity") -> (size(s)=w4274:i32)
            n3255 = Greater Than 0?(x=w4274) -> (x > 0?=w4273:bool)
            n3256 = call "Instrument fgv uno.vi"("Enum"=T28."WRITE", "error in (no error) 2"=w4277, "WriteCC1"="WriteHumidity", "INPUT"=w4276) -> ("error"=w4285:errorcluster, "WriteCC1 2"=w4275:string[], "output"=w4284:T17)  [unwired: 5 in]
            n3257 = case shown="True" w4273 {
              tunnel: w4275 -> [_ w4291]
              frame False {
              }
              frame True {
                n3258 = local write "WriteHumidity"(w4291) -> ()
              }
            }
            n3259 = case shown="No Error" w4285 {
              selector: w4285 -> [w4292 w4295]
              tunnel: w4284 -> [w4293 w4300]
              tunnel: [w4293 w4299] -> w4282
              tunnel: [w4292 w4297] -> w4283
              frame No Error {
              }
              frame Error {
                n3260 = call <vilib>:"Clear Errors.vi"("error in (no error)"=w4295) -> ("error out"=w4294:errorcluster)  [unwired: 5 in, 1 out]
                n3261 = call "Instrument fgv uno.vi"("Enum"=T28."ERROR INIT", "error in (no error) 2"=w4294, "INPUT"=w4300) -> ("error"=w4298:errorcluster, "output"=w4299:T17)  [unwired: 6 in, 1 out]
                n3262 = call <vilib>:"Clear Errors.vi"("error in (no error)"=w4298) -> ("error out"=w4297:errorcluster)  [unwired: 5 in, 1 out]
              }
            }
            n3263 = Unbundle By Name(w4282) -> ("LastCom"=→"LastCom Humidity":string, "Read Heave and Surge"=→"Read HUMIDITY":string)
          }
        }
        n3264 = Unbundle By Name(w4258) -> ("Heave COM Status 2"=w4259:bool, "Error Heave"=w4256:errorcluster, "Bytes at Heave Port"=→"Bytes at Humidity Port  2":dbl)  [unwired: 1 out]
        n3265 = Unbundle By Name(w4256) -> ("status"=→"Humidity Port":bool)
        n3266 = Not(x=w4259) -> (.not. x?=w4246:bool)
        n3267 = local read "Quit"() -> (w4250:bool)
        n3268 = local write "COM Status"(w4246) -> ()
        n3269 = Select(t=enum16{"init", "MAIN", "Panel Close"}."Panel Close", s=w4250, f=enum16{"init", "MAIN", "Panel Close"}."MAIN") -> (s? t:f=w4249:enum16{"init", "MAIN", "Panel Close"})
      }
      frame "Panel Close" {
      }
      frame Default {
      }
    }
  }
  n3270 = while {
    shift-right: [w4320] -> _
    shift-left: _ -> [w4321]
    shift-right: [w4318] -> _
    shift-left: T17 {"Read Heave and Surge"="", "Bytes at Heave Port"=0.0, "Heave and Surge COM Port:"="COM9", "Com Port 2"="COM7", "Residual Due"="", "Heave COM Status 2"=TRUE, "Heave COM Status"=TRUE, "Port 2"=TRUE, "Sway PPR"=6400.0, "Surge PPR"=6400.0, "Heave PPR"=6400.0, "Sway Pitch"=2.0, "Surge Pitch"=3.0, "Heave Pitch"=4.0, "Sway Pulses/mm"=320.0, "Surge Pulses/mm"=1600.0, "Heave Pulses/mm"=1600.0, "inner loop"=0.0, "Read Heave and Surge 2"="", "String 36"="", "Write S"=FALSE, "WriteCC1"=[""], "Heave COM Loop"=0, "LastCom"="", "EXIT"=FALSE, "Error Heave"={"status"=TRUE, "code"=-1073807343, "source"=""}} -> [w4317]
    shift-right: [w4315] -> _
    shift-left: enum16{"init", "MAIN", "Panel Close"}."init" -> [w4316]
    stop <- w4319 stop-if-true
    # "UNO CODE LOGIC"
    n3271 = case shown="\"MAIN\"" w4316 {
      tunnel: w4321 -> [w4335 w4352 w4410 w4412]
      tunnel: [w4329 w4358 w4410 w4412] -> w4320
      tunnel: [_ _ TRUE _] -> w4319
      tunnel: [w4325 w4356 w4408 w4411] -> w4318
      tunnel: w4317 -> [w4332 w4351 w4408 w4411]
      tunnel: [enum16{"init", "MAIN", "Panel Close"}."MAIN" w4345 _ _] -> w4315
      frame "init" {
        n3272 = Bundle By Name(cluster=w4332, "Heave and Surge COM Port:"="C3 :") -> (w4331:T17)
        n3273 = call "Instrument fgv.vi"("Enum"=T28."INIT", "error in (no error) 2"=w4335, "INPUT"=w4331) -> ("error"=w4333:errorcluster, "output"=w4328:T17)  [unwired: 6 in, 1 out]
        n3274 = case shown="Error" w4333 {
          selector: w4333 -> [w4337 _]
          tunnel: [w4337 w4341] -> w4329
          tunnel: w4328 -> [w4336 w4339]
          tunnel: [w4336 w4338] -> w4326
          frame No Error {
          }
          frame Error {
            n3275 = call "Instrument fgv.vi"("Enum"=T28."ERROR INIT", "INPUT"=w4339) -> ("error"=w4342:errorcluster, "output"=w4338:T17)  [unwired: 7 in, 1 out]
            n3276 = call <vilib>:"Clear Errors.vi"("error in (no error)"=w4342) -> ("error out"=w4341:errorcluster)  [unwired: 5 in, 1 out]
          }
        }
        n3277 = local read "LastCom UNO"() -> (w4322:string)
        n3278 = Unbundle By Name(w4326) -> ("Heave COM Status 2"=→"Instrument Status":bool, "Error Heave"=→"Error":errorcluster)  [unwired: 1 out]
        n3279 = Bundle By Name(cluster=w4326, "LastCom"=w4322) -> (w4325:T17)
      }
      frame "MAIN" {
        n3280 = Unbundle By Name(w4351) -> ("Com Port 2"=w4360:refnum<visa-resource-name>)
        n3281 = local write "Com Port 4"(w4360) -> ()
        n3282 = local read "C3 :"() -> (w4349:refnum<visa-resource-name>)
        n3283 = Bundle By Name(cluster=w4351, "Heave and Surge COM Port:"=w4349) -> (w4350:T17)
        n3284 = Equal?(x=w4360, y=w4349) -> (x = y?=w4359:bool)
        n3285 = case shown="True" w4359 {
          tunnel: [w4364 w4381] -> w4358
          tunnel: w4352 -> [w4365 w4387]
          tunnel: w4350 -> [w4363 w4385]
          tunnel: [w4362 w4380] -> w4356
          frame False {
            n3286 = call <vilib>:"Clear Errors.vi"("error in (no error)"=w4365) -> ("error out"=w4361:errorcluster)  [unwired: 5 in, 1 out]
            n3287 = call "Instrument fgv.vi"("Enum"=T28."ERROR INIT", "error in (no error) 2"=w4361, "INPUT"=w4363) -> ("error"=w4367:errorcluster, "output"=w4362:T17)  [unwired: 6 in, 1 out]
            n3288 = call <vilib>:"Clear Errors.vi"("error in (no error)"=w4367) -> ("error out"=w4364:errorcluster)  [unwired: 5 in, 1 out]
          }
          frame True {
            n3289 = call "Instrument fgv.vi"("Enum"=T28."READ", "error in (no error) 2"=w4387, "INPUT"=w4385) -> ("error"=w4386:errorcluster, "output"=w4378:T17)  [unwired: 6 in, 1 out]
            n3290 = Bundle By Name(cluster=w4378, "String 36"="WRITE UNO") -> (w4377:T17)
            n3291 = case shown="True" "Write S" {
              selector: "Write S" -> [_ w4407]
              tunnel: w4386 -> [w4400 w4406]
              tunnel: [w4400 w4405] -> w4375
              tunnel: w4377 -> [w4399 w4402]
              tunnel: [w4399 w4401] -> w4374
              frame False {
              }
              frame True {
                n3292 = Not(x=w4407) -> (.not. x?=w4403:bool)
                n3293 = local write "Write S"(w4403) -> ()
                n3294 = call "Instrument fgv.vi"("Enum"=T28."MANUAL WRITE", "error in (no error) 2"=w4406, "INPUT"=w4402) -> ("error"=w4405:errorcluster, "output"=w4401:T17)  [unwired: 6 in, 1 out]
              }
            }
            n3295 = Array Size(array="Write UNO") -> (size(s)=w4372:i32)
            n3296 = Greater Than 0?(x=w4372) -> (x > 0?=w4371:bool)
            n3297 = call "Instrument fgv.vi"("Enum"=T28."WRITE", "error in (no error) 2"=w4375, "WriteCC1"="Write UNO", "INPUT"=w4374) -> ("error"=w4383:errorcluster, "WriteCC1 2"=w4373:string[], "output"=w4382:T17)  [unwired: 5 in]
            n3298 = case shown="True" w4371 {
              tunnel: w4373 -> [_ w4389]
              frame False {
              }
              frame True {
                n3299 = local write "Write UNO"(w4389) -> ()
              }
            }
            n3300 = case shown="Error" w4383 {
              selector: w4383 -> [w4390 w4393]
              tunnel: w4382 -> [w4391 w4398]
              tunnel: [w4391 w4397] -> w4380
              tunnel: [w4390 w4395] -> w4381
              frame No Error {
              }
              frame Error {
                n3301 = call <vilib>:"Clear Errors.vi"("error in (no error)"=w4393) -> ("error out"=w4392:errorcluster)  [unwired: 5 in, 1 out]
                n3302 = call "Instrument fgv.vi"("Enum"=T28."ERROR INIT", "error in (no error) 2"=w4392, "INPUT"=w4398) -> ("error"=w4396:errorcluster, "output"=w4397:T17)  [unwired: 6 in, 1 out]
                n3303 = call <vilib>:"Clear Errors.vi"("error in (no error)"=w4396) -> ("error out"=w4395:errorcluster)  [unwired: 5 in, 1 out]
              }
            }
            n3304 = Unbundle By Name(w4380) -> ("LastCom"=→"LastCom UNO":string, "Read Heave and Surge"=→"Read UNO":string)
          }
        }
        n3305 = Unbundle By Name(w4356) -> ("Heave COM Status 2"=w4357:bool, "Heave COM Status"=w4344:bool, "Error Heave"=w4354:errorcluster, "Bytes at Heave Port"=→"Bytes at Humidity Port":dbl)
        n3306 = Unbundle By Name(w4354) -> ()  [unwired: 1 out]
        n3307 = Not(x=w4344) -> (.not. x?=w4353:bool)
        n3308 = local write "Error"(w4354) -> ()
        n3309 = Not(x=w4357) -> (.not. x?=w4343:bool)
        n3310 = local write "Instrument Status"(w4353) -> ()
        n3311 = local write "Port 1a"(w4344) -> ()
        n3312 = local read "Quit"() -> (w4346:bool)
        n3313 = local write "COM Status"(w4343) -> ()
        n3314 = Select(t=enum16{"init", "MAIN", "Panel Close"}."Panel Close", s=w4346, f=enum16{"init", "MAIN", "Panel Close"}."MAIN") -> (s? t:f=w4345:enum16{"init", "MAIN", "Panel Close"})
      }
      frame "Panel Close" {
      }
      frame Default {
      }
    }
  }
  n3315 = while {
    stop <- w4438 stop-if-true
    n3316 = local read "Read HUMIDITY"() -> (w4413:string)
    n3317 = call <vilib>:"High Resolution Polling Wait.vi"("seconds to wait"=0.05) -> ()  [unwired: 10 in, 1 out]
    n3318 = Spreadsheet String To Array(delimiter (Tab)=",", format string="", spreadsheet string=w4413, array type (2D Dbl)=string[] []) -> (array=w4433:string[])
    n3319 = for {
      tunnel: w4433 -> [w4443] mode=indexing
      tunnel: string[] ["STATE;", "SET;", "RH;", "T;", "AMB_RH;", "AMB_T;", "PUMP;", "FAN_IN;", "FAN_OUT;", "DEHUM;", "CURRENT;", "STALL;"] -> [w4442] mode=indexing
      tunnel: [w4441] -> w4432 mode=indexing
      n3320 = Match Pattern(string=w4443, regular expression=w4442) -> (after substring=w4441:string)  [unwired: 1 in, 3 out]
    }
    n3321 = Index Array(array=w4432) -> (element #1=→"STATE :":string, element #2=→"SET :":string, element #3=w4421:string, element #4=→"T :":string, element #5=w4419:string, element #6=→"AMB_T :":string, element #7=→"PUMP :":string, element #8=→"FAN_IN :":string, element #9=→"FAN_OUT :":string, element #10=→"DEHUM :":string, element #11=→"CURRENT :":string, element #12=→"STALL :":string)  [unwired: 12 in]
    "RH :" <- w4421
    "AMB_RH :" <- w4419
    n3322 = Fract/Exp String To Number(string=w4421) -> (number=w4414:dbl)  [unwired: 3 in, 1 out]
    n3323 = Fract/Exp String To Number(string=w4419) -> (number=w4418:dbl)  [unwired: 3 in, 1 out]
    n3324 = local write "Ambient Humidity :"(w4418) -> ()
    n3325 = Equal?(x=w4414, y=0.0) -> (x = y?=w4416:bool)
    n3326 = case shown="True" w4416 {
      tunnel: [w4439 w4440] -> w4415
      tunnel: w4414 -> [w4439 _]
      frame False {
        (unwired) 0.0
        "Humidity temp" <- w4439
      }
      frame True {
        n3327 = local read "Humidity temp"() -> (w4440:dbl)
      }
    }
    "RH Numeric:" <- w4415
    n3328 = local read "Quit"() -> (w4438:bool)
  }
